vi "指定范围的随机数(demo).vi"(0 "上限 (1.00)":dbl=1.0 format="%.2f", 1 "下限 (0.00)":dbl format="%.2f") -> (4 "随机数":dbl format="%.2f")   [LabVIEW 2012]
doc: "功能：\n\n产生指定范围的<b>随机数</b>。\n\n\n\n\n\ncsxcs_366创建"
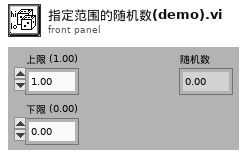
[diagram p1: front panel]
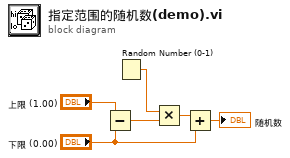
[diagram p0: block diagram]
diagram:
  n1 = Subtract(x="上限 (1.00)", y="下限 (0.00)") -> (x-y=w3:dbl)
  n2 = Random Number (0-1)() -> (number: 0 to 1=w6:dbl)
  n3 = Multiply(x=w6, y=w3) -> (x*y=w1:dbl)
  n4 = Add(x=w1, y="下限 (0.00)") -> (x+y=→"随机数":dbl)
